vi "SetCurrentScreen.vi"(8 "error in (no error)":errorcluster, 11 "Game in":refnum<class "Game.lvclass">) -> (0 "error out":errorcluster, 3 "Game out":refnum<class "Game.lvclass">)   [LabVIEW 2019, in "RT_Game.lvlib" / "Game.lvclass"]
uses:
  Game.lvclass
  Coordinate.ctl
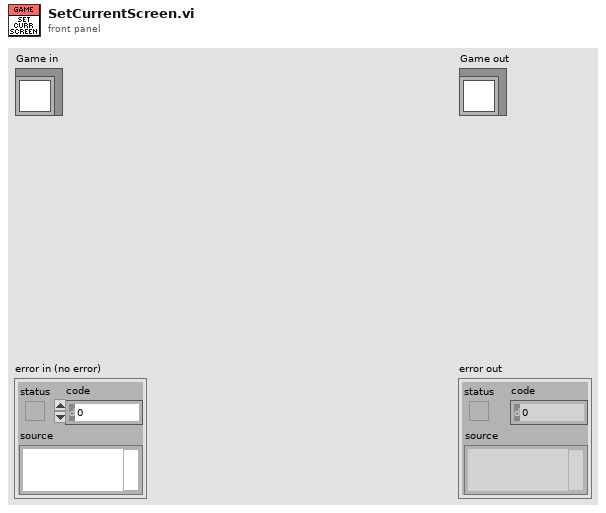
[diagram p1: front panel]
types:
  T1 = typedef "RT_Game.lvlib/Game.lvclass/Coordinate.ctl" = cluster{"x":dbl, "y":dbl}
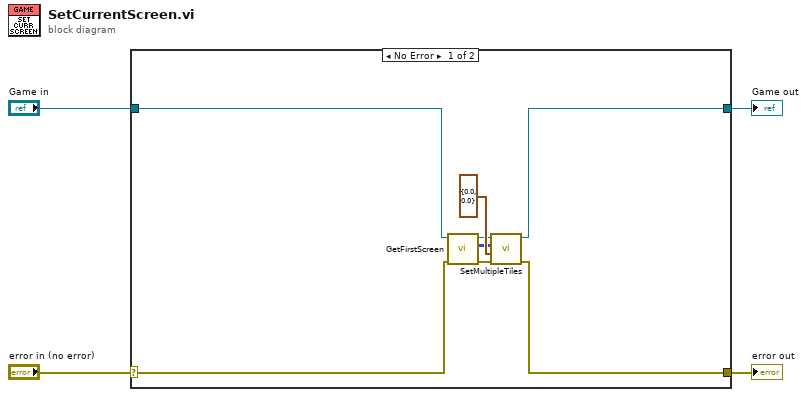
[diagram p0: block diagram]
diagram:
  n1 = case shown="No Error" "error in (no error)" {
    selector: "error in (no error)" -> [w6 w14]
    tunnel: [w5 w14] -> w3
    tunnel: [w8 w13] -> w1
    tunnel: "Game in" -> [w7 w13]
    frame No Error {
      n2 = call-dynamic "GetFirstScreen.vi"("error in (no error)"=w6, "Game in"=w7) -> ("error out"=w9:errorcluster, "Array"=w11:u32[][], "Game out"=w10:refnum<class "Game.lvclass">)  [unwired: 7 in]
      n3 = call "SetMultipleTiles.vi"("error in (no error)"=w9, "Position"=T1 {"x"=0.0, "y"=0.0}, "TileCodes"=w11, "Game in"=w10) -> ("error out"=w5:errorcluster, "Game out"=w8:refnum<class "Game.lvclass">)  [unwired: 6 in]
    }
    frame Error {
    }
  }
  "error out" <- w3
  "Game out" <- w1
